vi "sistema_labview.vi"() -> ()   [LabVIEW 2026]
uses:
  <vilib>/Instr/_visa.llb/VISA Flush IO Buffer Mask.ctl
  <vilib>/Instr/_visa.llb/VISA Configure Serial Port (Instr).vi
  tektronix_dpo_mso_2000_4000_series 2/Tektronix DPO MSO 2000 4000 Series/Public/Data/Read (Single Waveform).vi
  <vilib>/express/express analysis/Spectral/Block/exnSpectralBlock spectral measurements RMS poly.vi
  <vilib>/express/express analysis/Spectral/Block/exnSpectralBlock spectral measurements RMS DDT.vi
  <vilib>/express/express analysis/Spectral/XNode/ExpressSpectralMeasurementsBlockNode.xnode
  tektronix_dpo_mso_2000_4000_series 2/Tektronix DPO MSO 2000 4000 Series/Tektronix DPO MSO 2000 4000 Series.lvlib
panel:
  in  "Record":bool
  in  "Filename 2":path=path "test.xlsx" caption="Filename"
  in  "Channel (0: Channel 1)":u16(ring) items=["Channel 1", "Channel 2", "Channel 3", "Channel 4", "Math", "Reference 1", "Reference 2", "Reference 3", "Reference 4"]
  in  "VISA Resource Name 2":refnum<visa-resource-name>
  out "Com Arduino OK":bool
  in  "VISA resource name":refnum<visa-resource-name>
  out "Motor 1 Round":dbl
  out "Motor 2 Round":dbl
  in  "Resolution (passo/mm)":dbl
  in  "Run Beam":bool
  in  "?":bool=TRUE
  out "Axis 2 Offset":dbl
  out "Axis 1 Offset":dbl
  out "Move Motor 1 (x)":dbl=-3.0
  out "Move Motor 2 (z)":dbl=1.0
  out "Scan Loop":u32=9
  out "Imaging Locations (z,x)":dbl[][](array[numeric])=[[5.0, -5.0], [3.0, -5.0], [1.0, -5.0], [-1.0, -5.0], [-3.0, -5.0], [-5.0, -5.0], [-5.0, -3.0], [-3.0, -3.0], [-1.0, -3.0], [1.0, -3.0], [3.0, -3.0], [5.0, -3.0], [5.0, -1.0], [3.0, -1.0], [1.0, -1.0], [-1.0, -1.0], [-3.0, -1.0], [-5.0, -1.0], [-5.0, 1.0], [-3.0, 1.0], [-1.0, 1.0], [1.0, 1.0], [3.0, 1.0], [5.0, 1.0], [5.0, 3.0], [3.0, 3.0], [1.0, 3.0], [-1.0, 3.0], [-3.0, 3.0], [-5.0, 3.0]]
  out "Graph Locations (x,z)":u32[][](array[numeric])
  out "Scanned Data positive":dbl[][](array[numeric])
  out "Scanned Data negative":dbl[][](array[numeric])
  out "Axis 2 Step":dbl=10.0
  out "Axis 1 Step":dbl
  out "Placement":dbl[](array[numeric])
  out "Beam Map Execution (%)":dbl(knob)=0.3 scale=0.0..1.0
  in  "Axis 2 Divisions":u32=5
  in  "Axis 1 Divisions":u32=5
  in  "Axis 1 Distance x(mm)":dbl=10.0
  in  "Axis 2 Distance z(mm)":dbl=10.0
  out "initialized array":dbl[][](array[numeric])
  out "output array":dbl[][](array[numeric])
  out "Intensity Graph":dbl[][](graph)
  out "Z inicial (PACE)":i32
  out "X inicial (PACE)":i32
  in  "X min FFT (kHz)":dbl
  in  "X max FFT (MHz)":dbl=4000.0
  in  "Y max scope (V)":dbl=1.0
  in  "Y min scope (V)":dbl=-1.0
  in  "X max scope (us)":dbl=100.0
  in  "X min scope (us)":dbl
  in  "Lower Cut-Off":dbl=100.0
  in  "Activate Filter":bool
  out "Frequency Spectrum":dynamicdata(graph)
  out "Osciloscopio":dynamicdata(graph)
  in  "offset":dbl
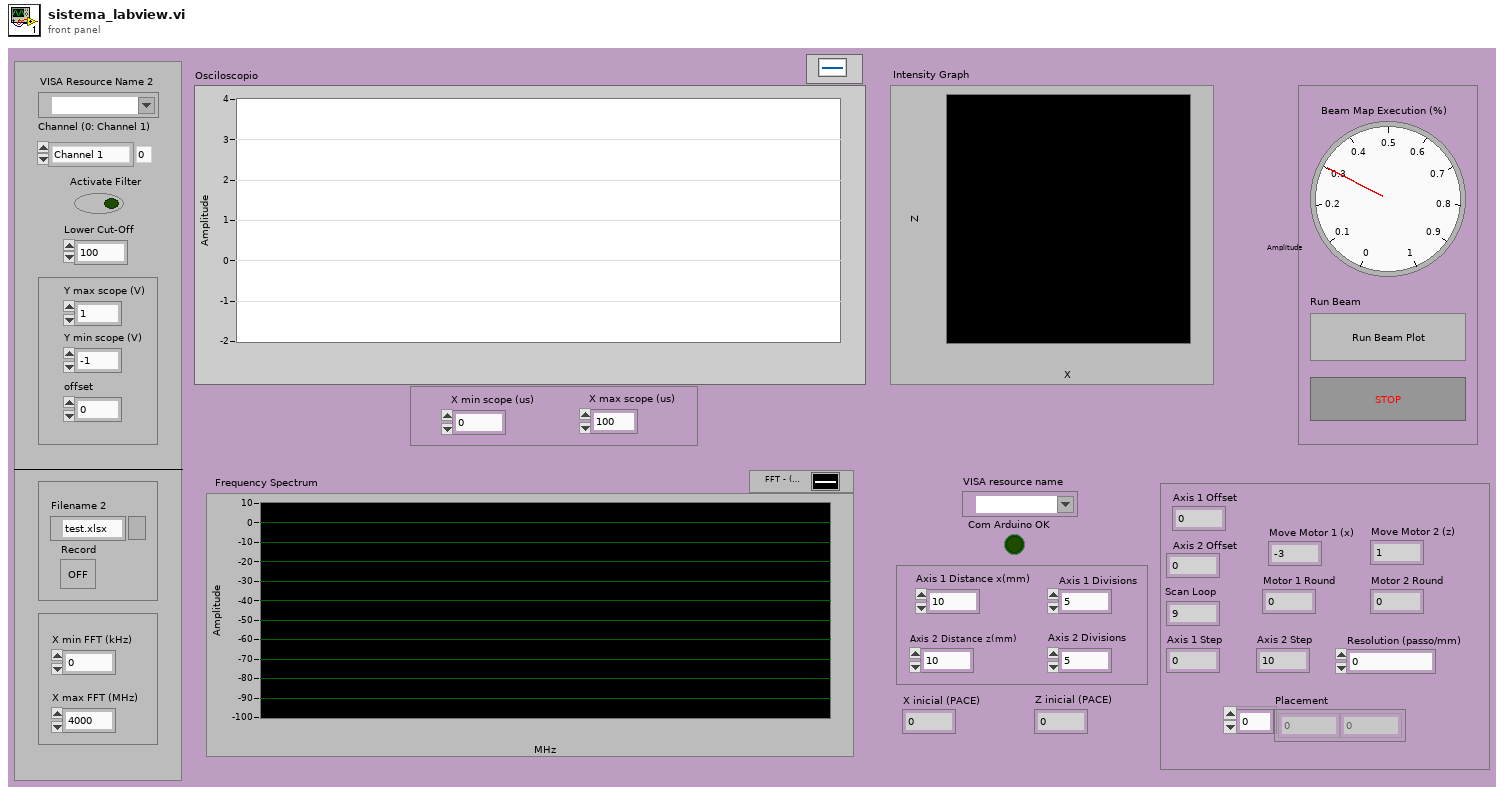
[diagram p1: front panel]
types:
  T1 = typedef "VISA Flush IO Buffer Mask.ctl" = u16
  T2 = cluster{"averaging mode":u16, "weighting mode":u16, "number of averages":u32}
  T3 = cluster{"dB On (F)":bool, "unwrap phase (F)":bool, "convert to degree (F)":bool}
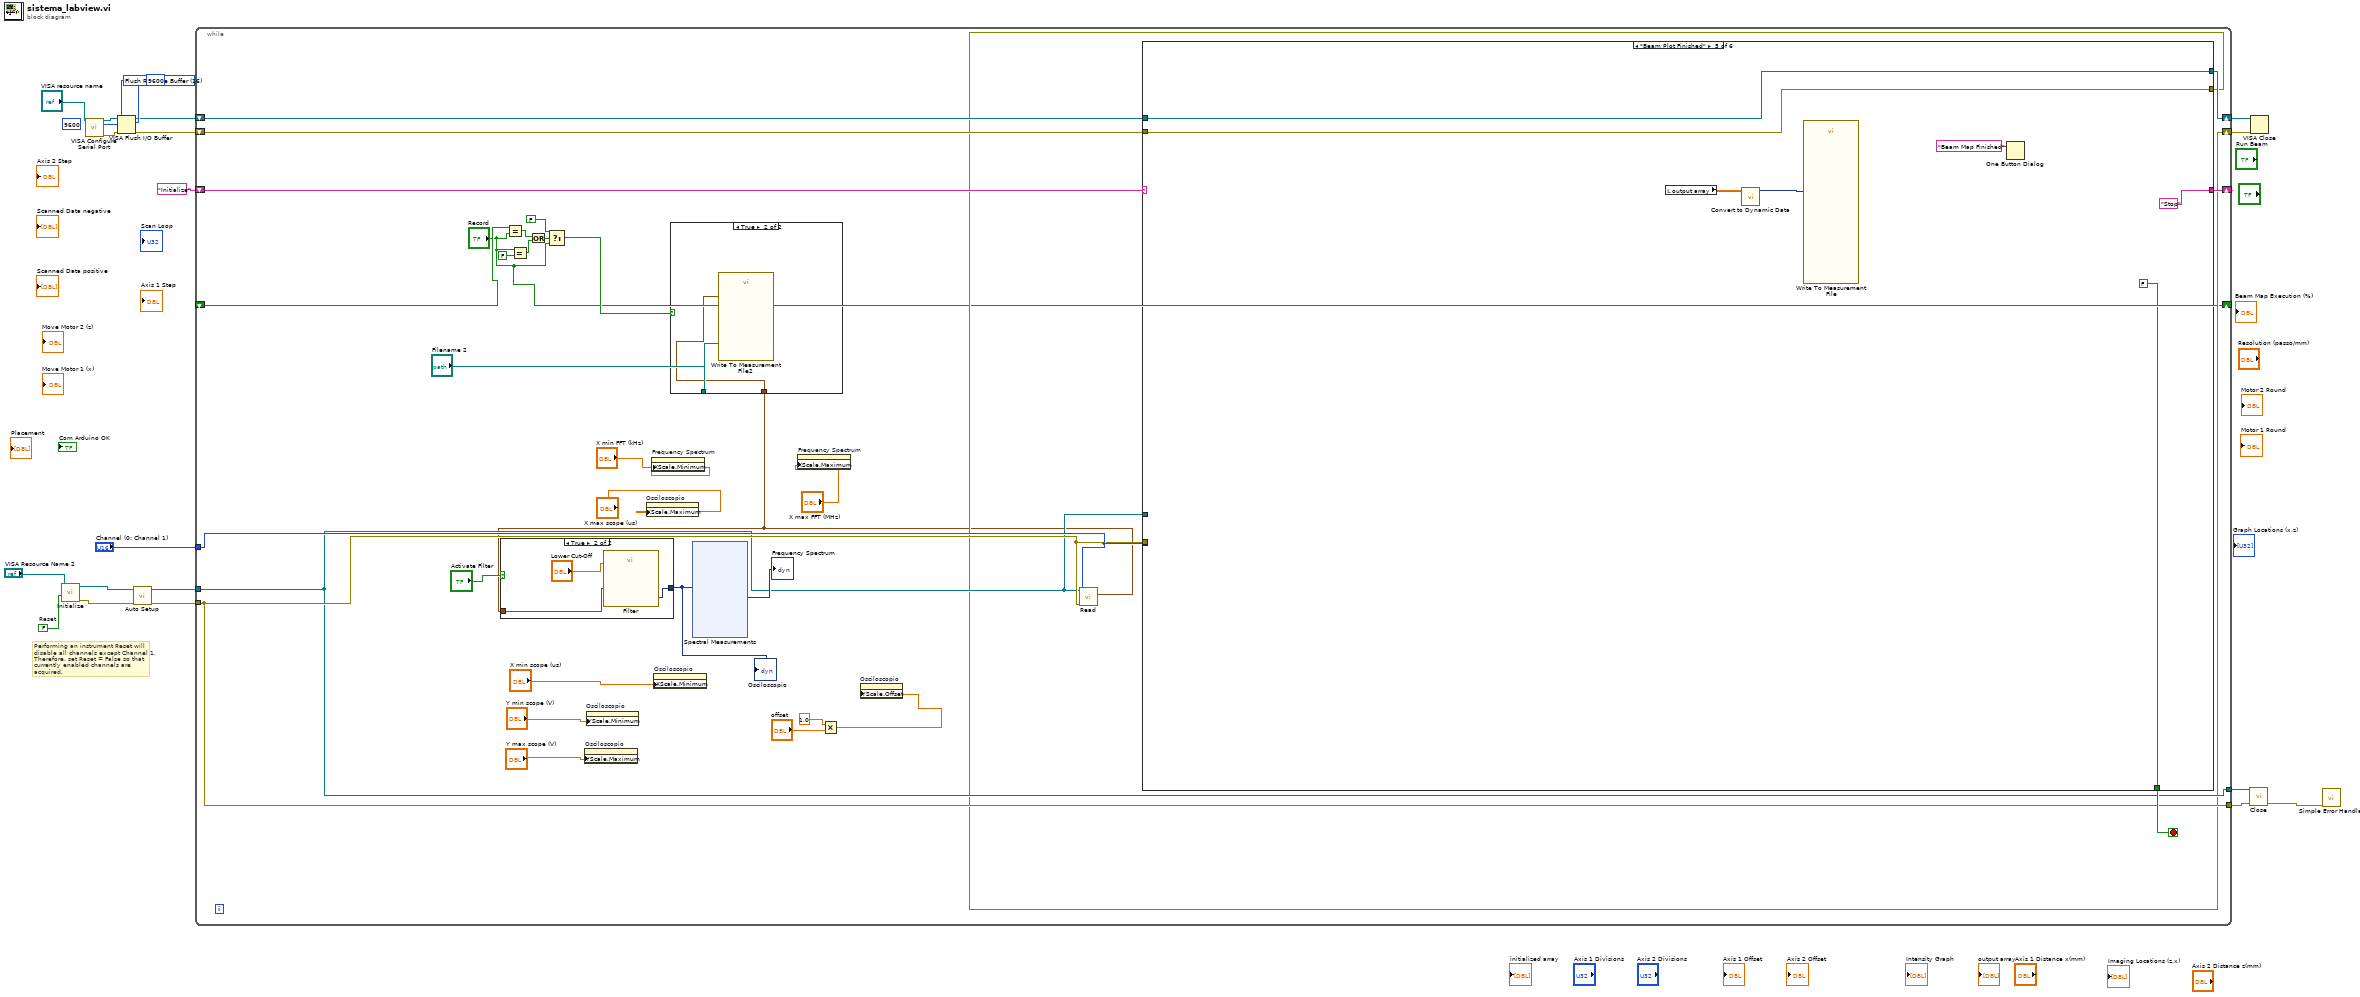
[diagram p0: block diagram]
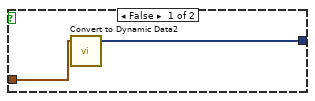
[diagram p3: hidden frame]
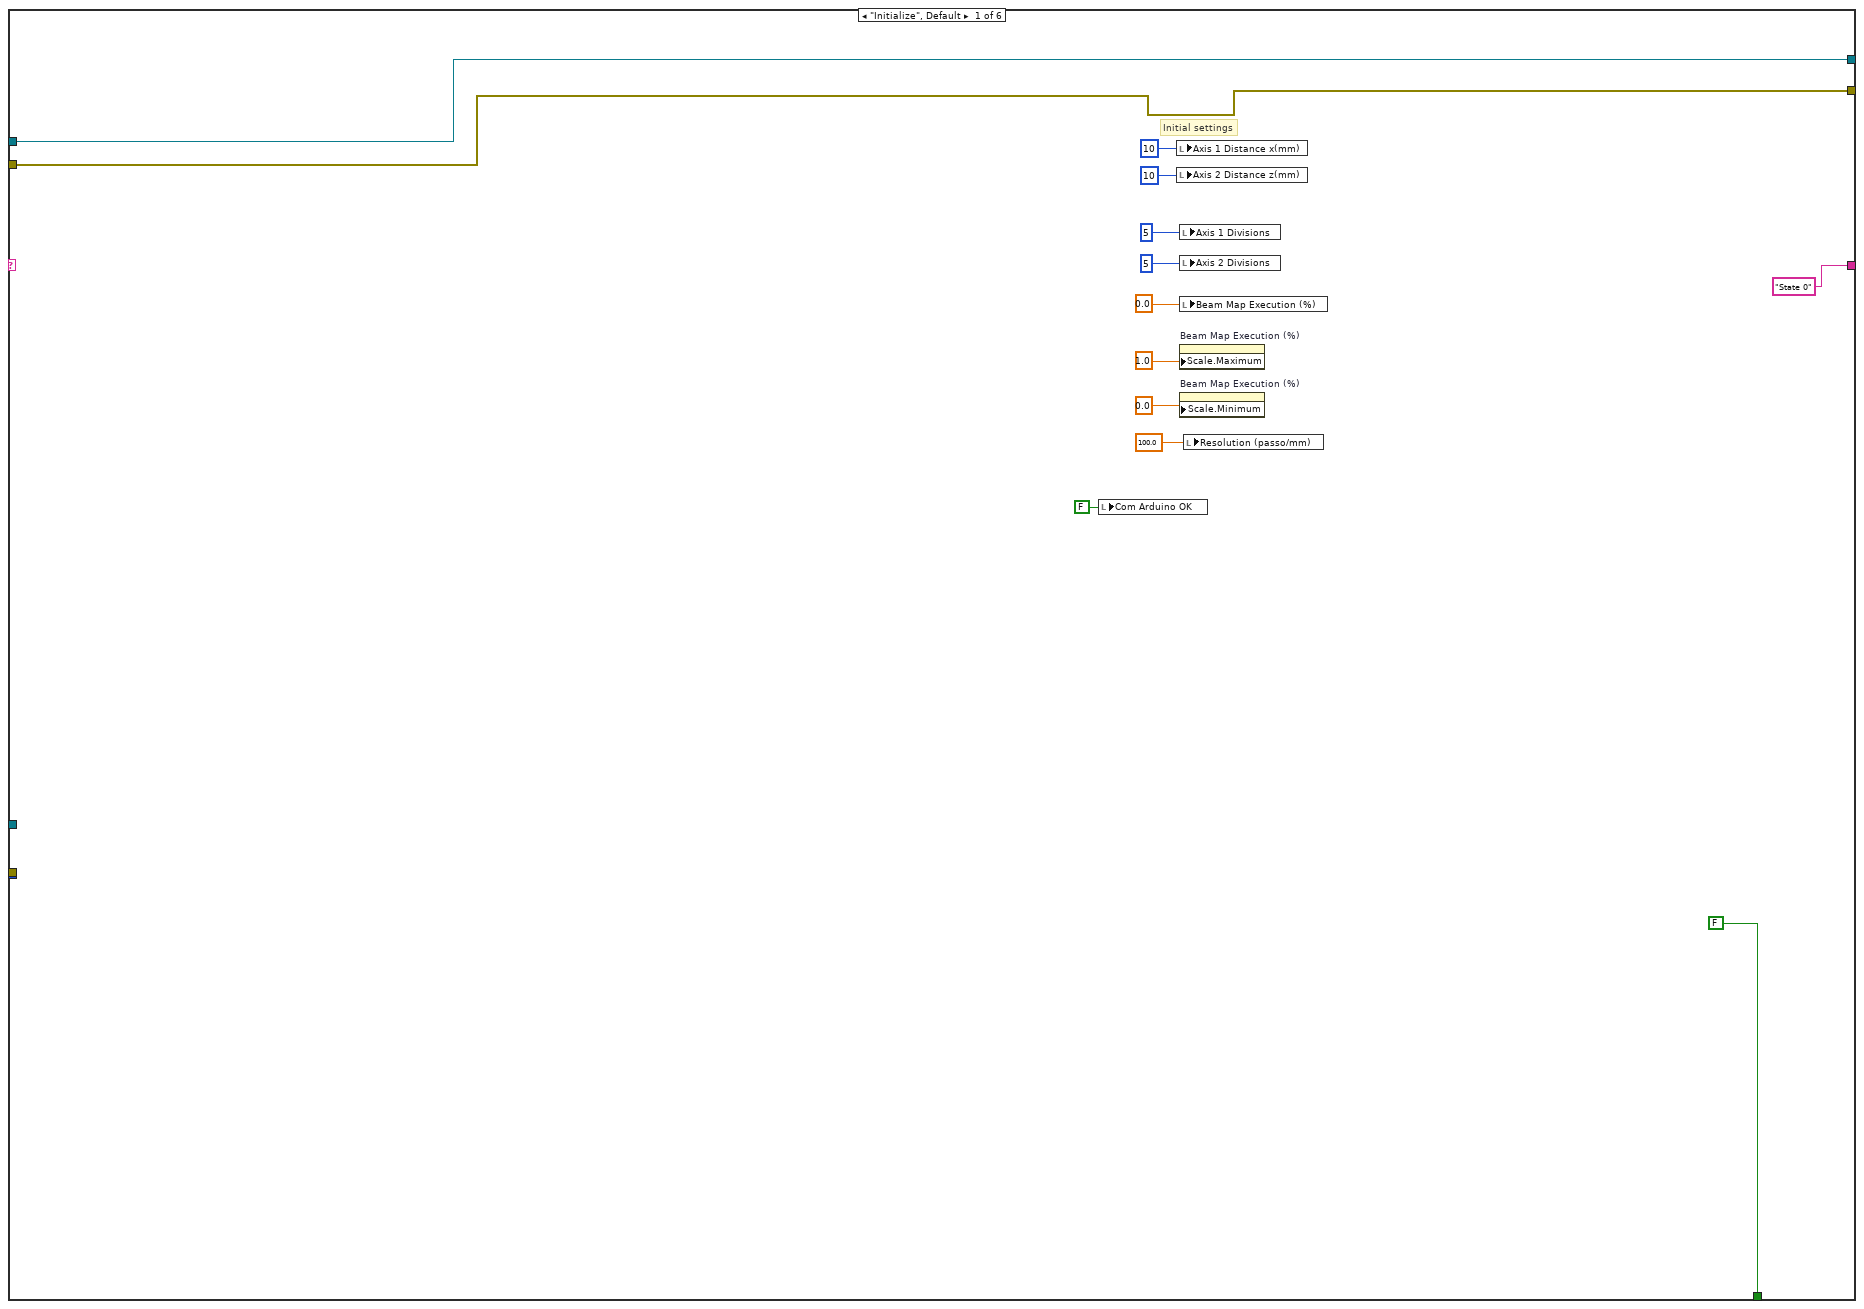
[diagram p4: hidden frame]
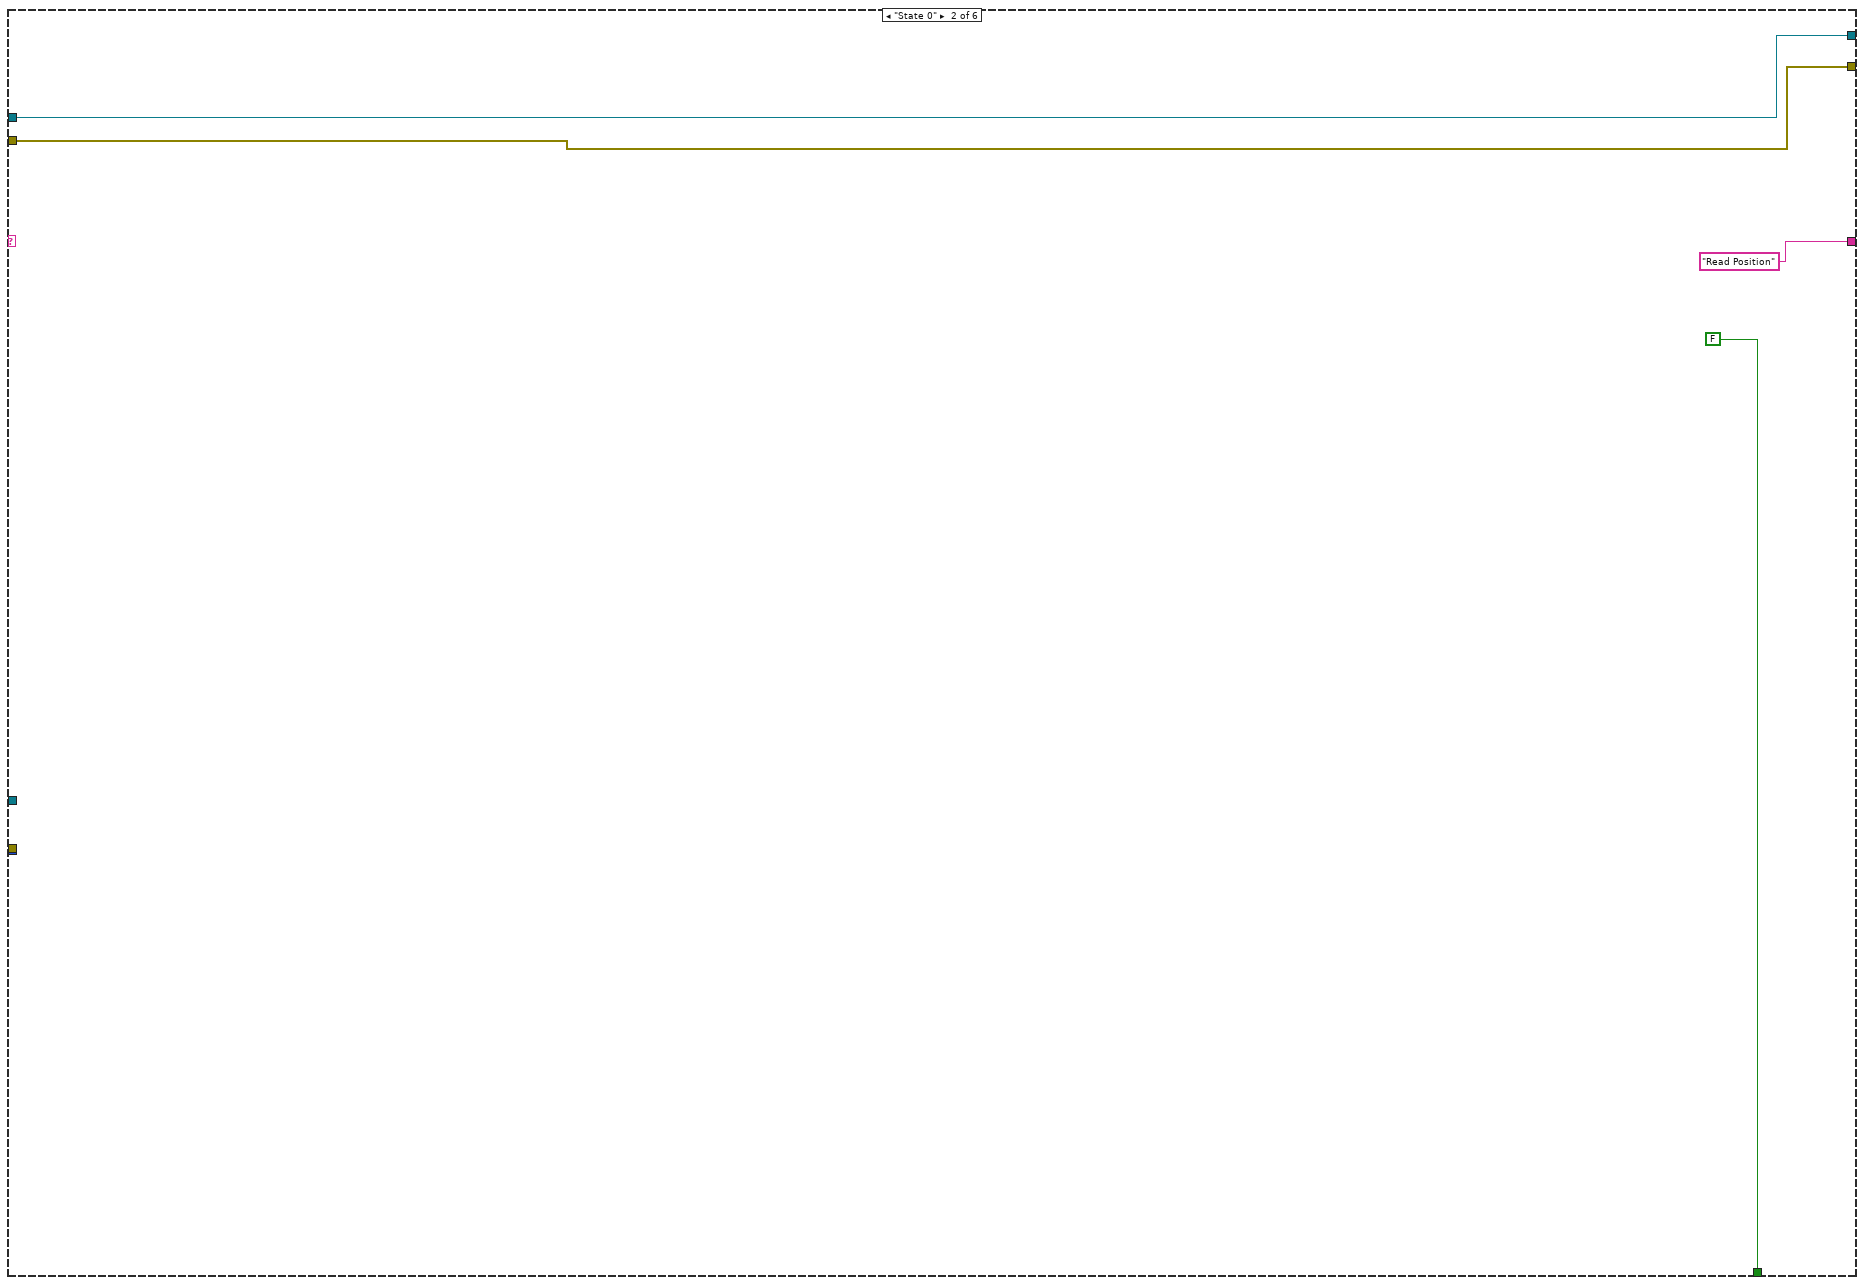
[diagram p5: hidden frame]
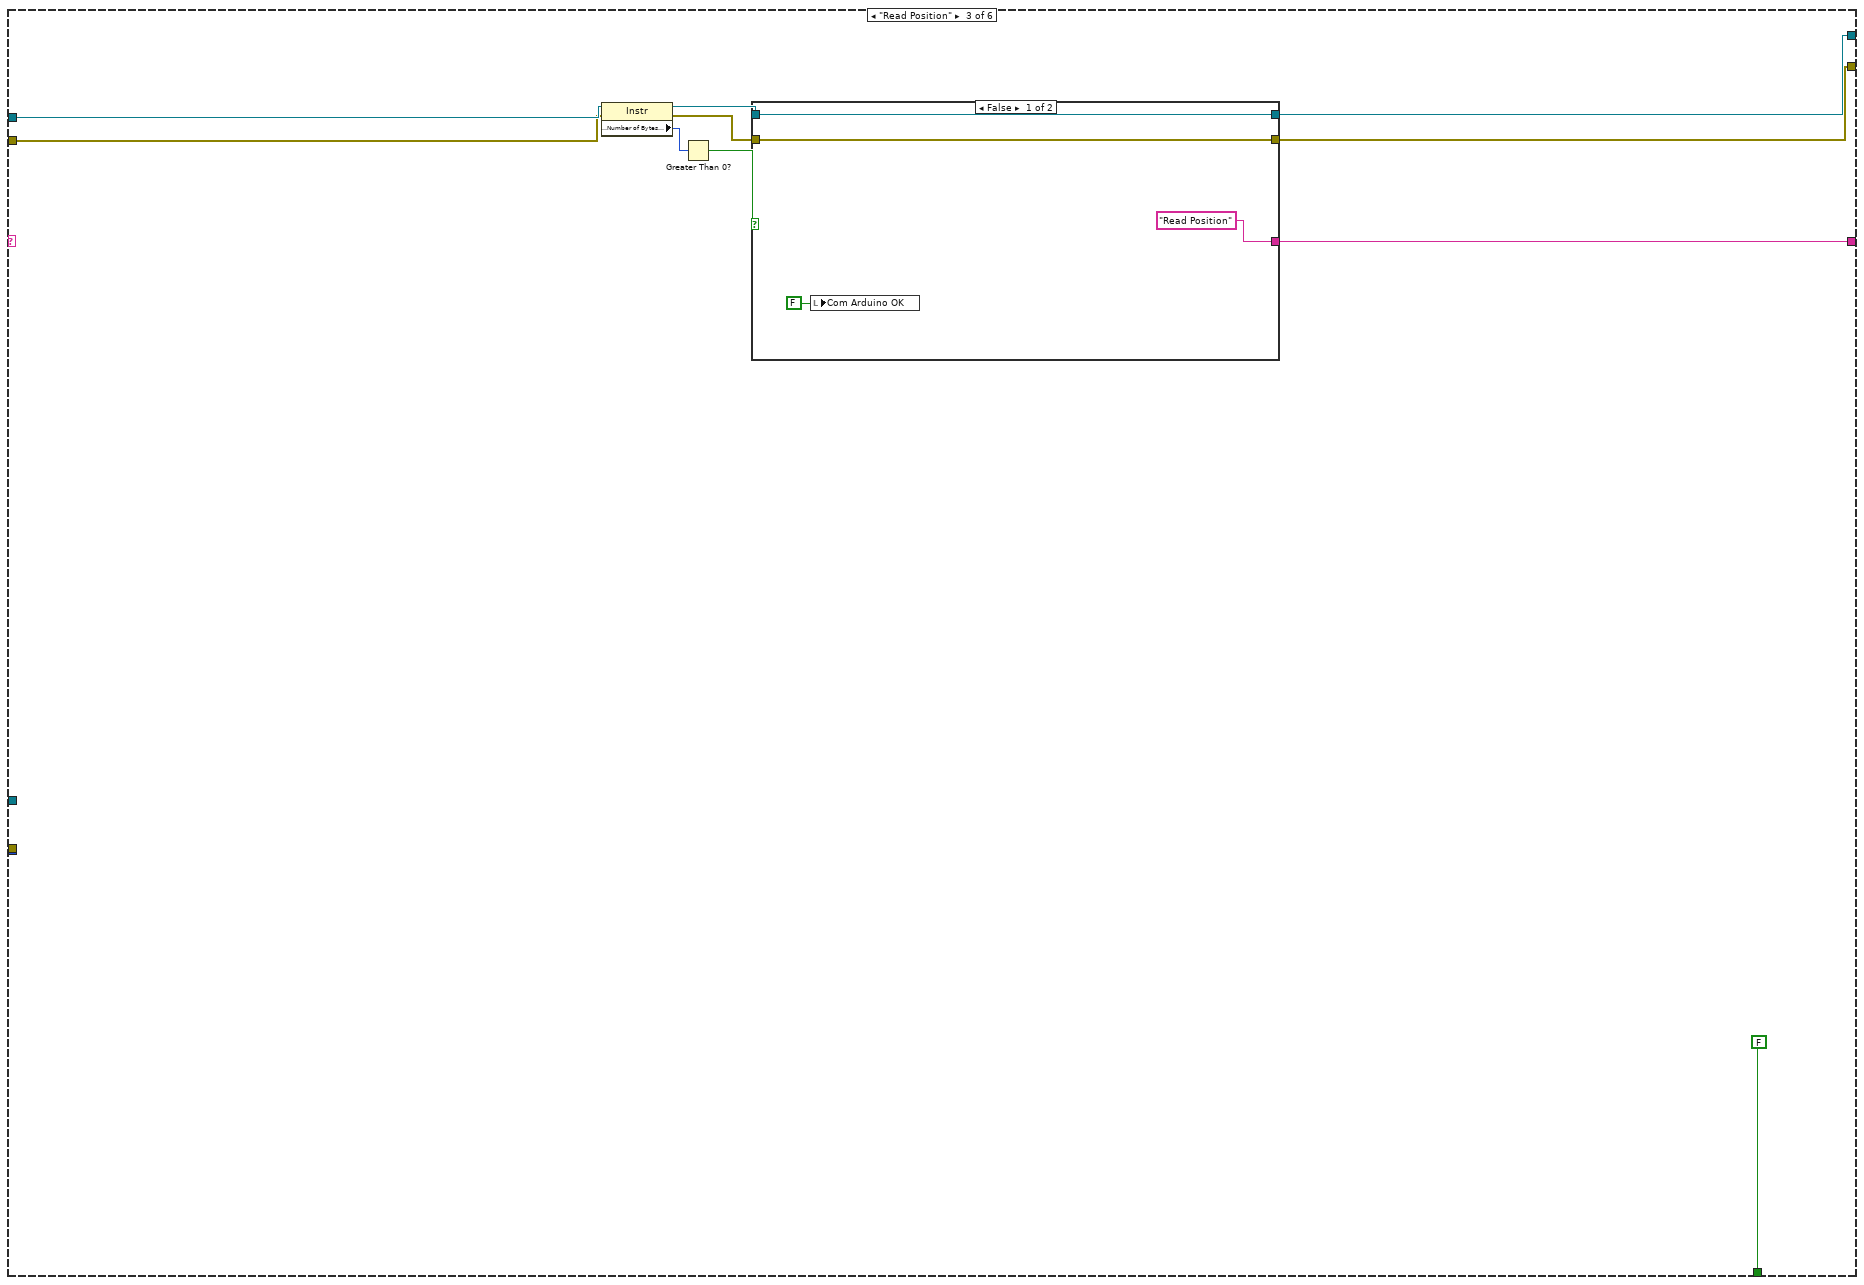
[diagram p6: hidden frame]
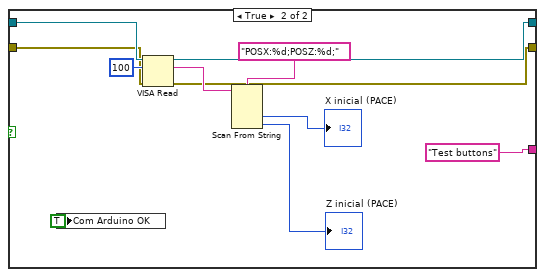
[diagram p7: hidden frame]
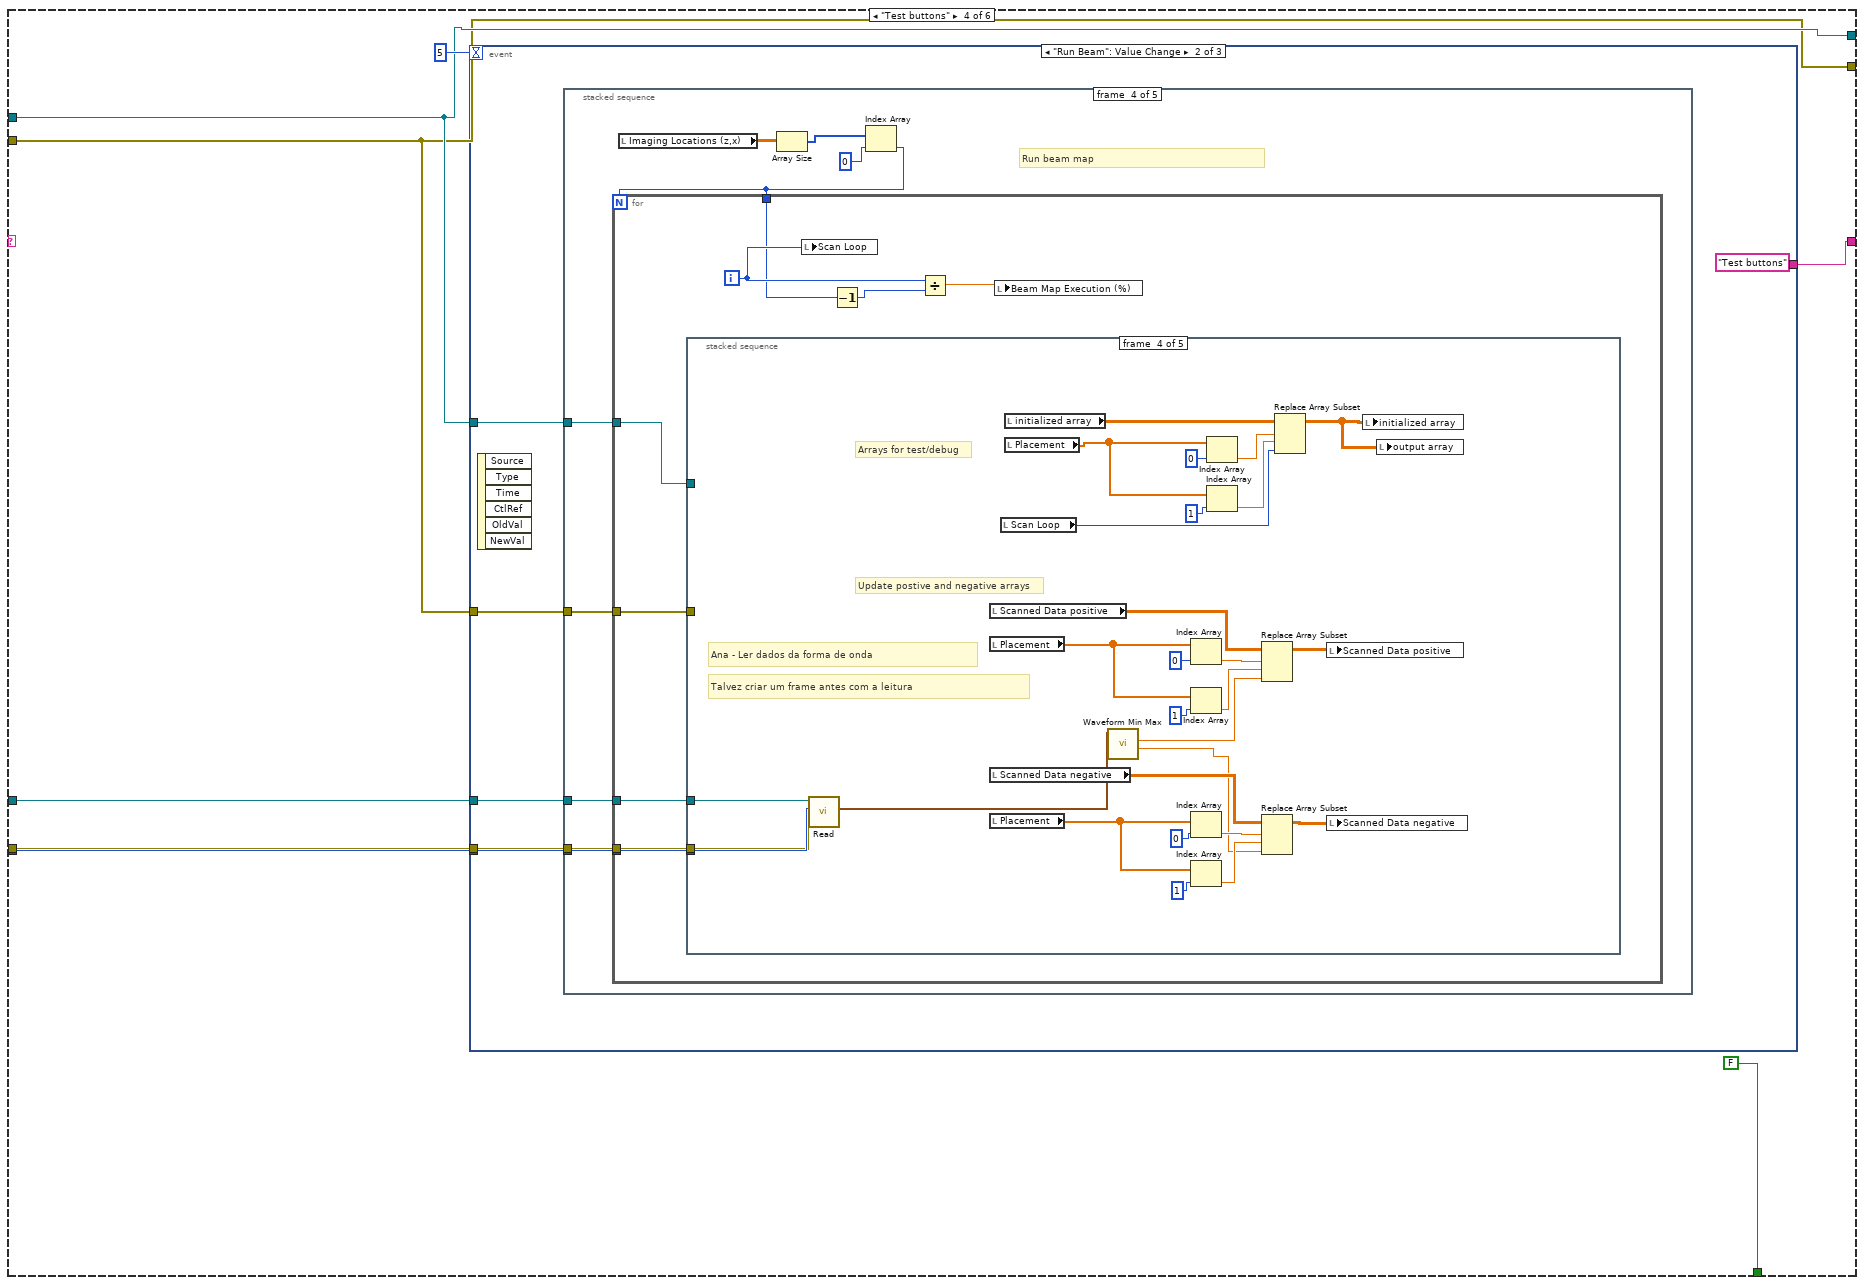
[diagram p8: hidden frame]
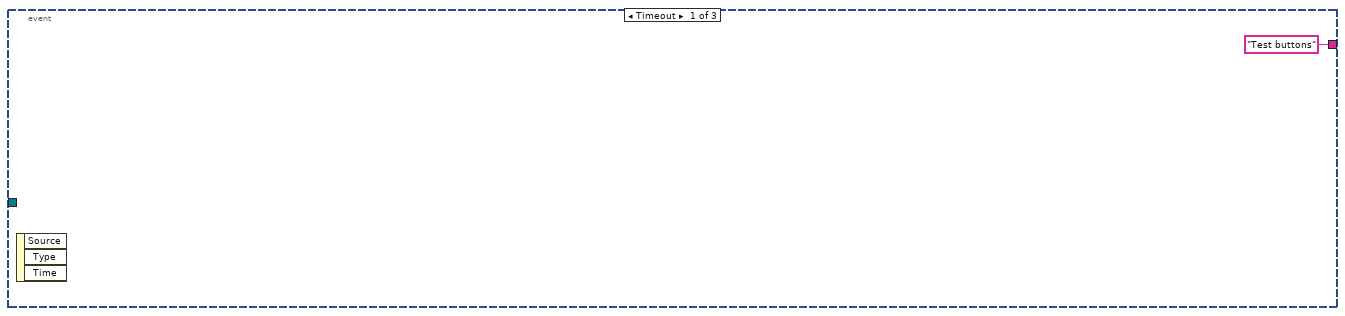
[diagram p9: hidden frame]
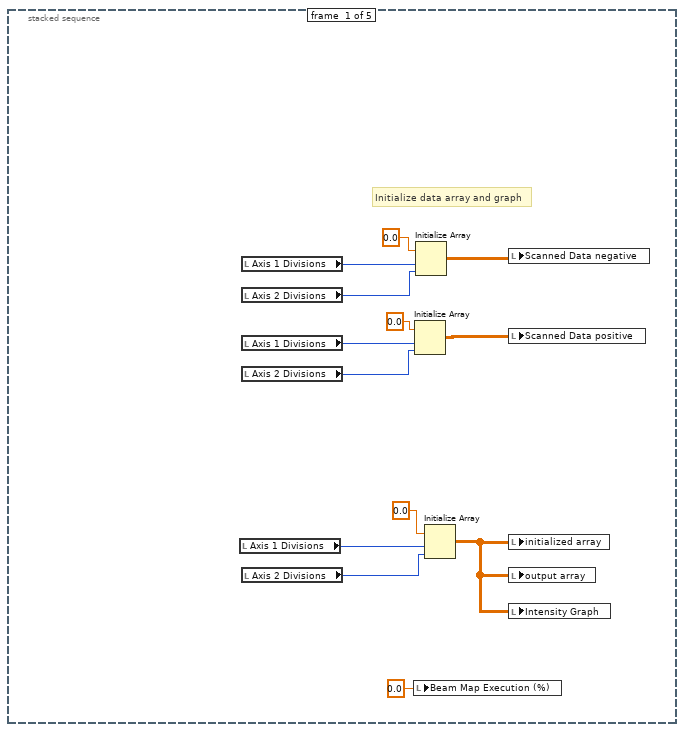
[diagram p10: hidden frame]
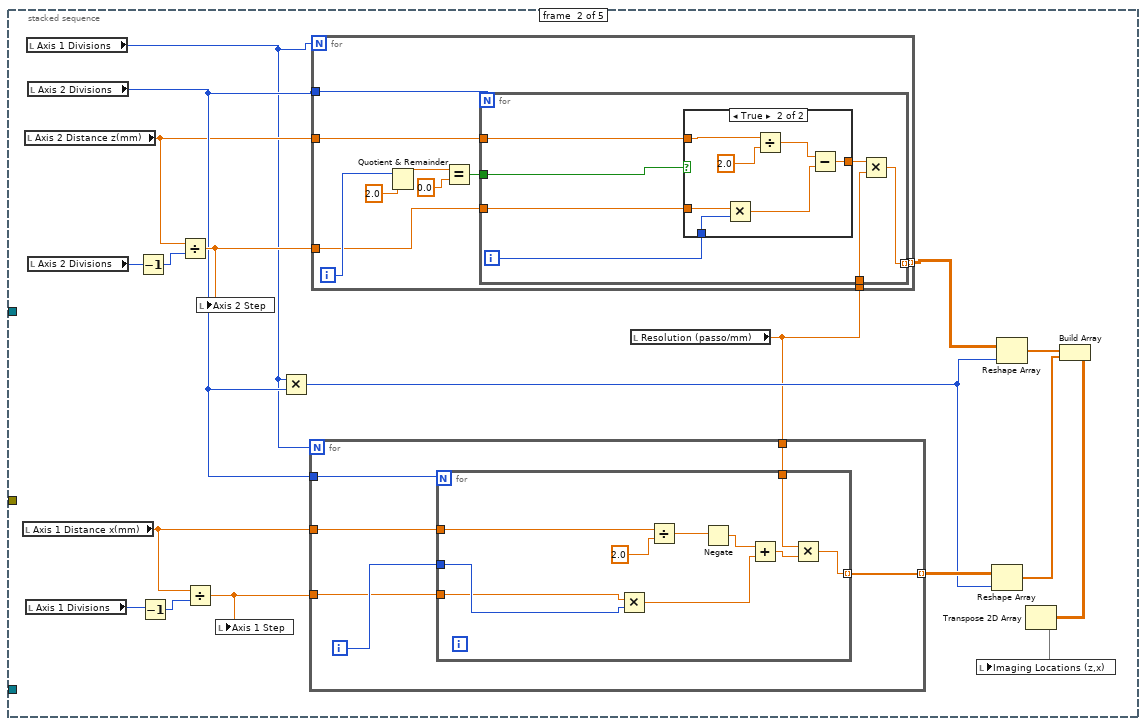
[diagram p11: hidden frame]
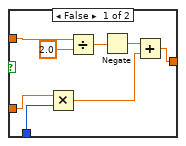
[diagram p12: hidden frame]
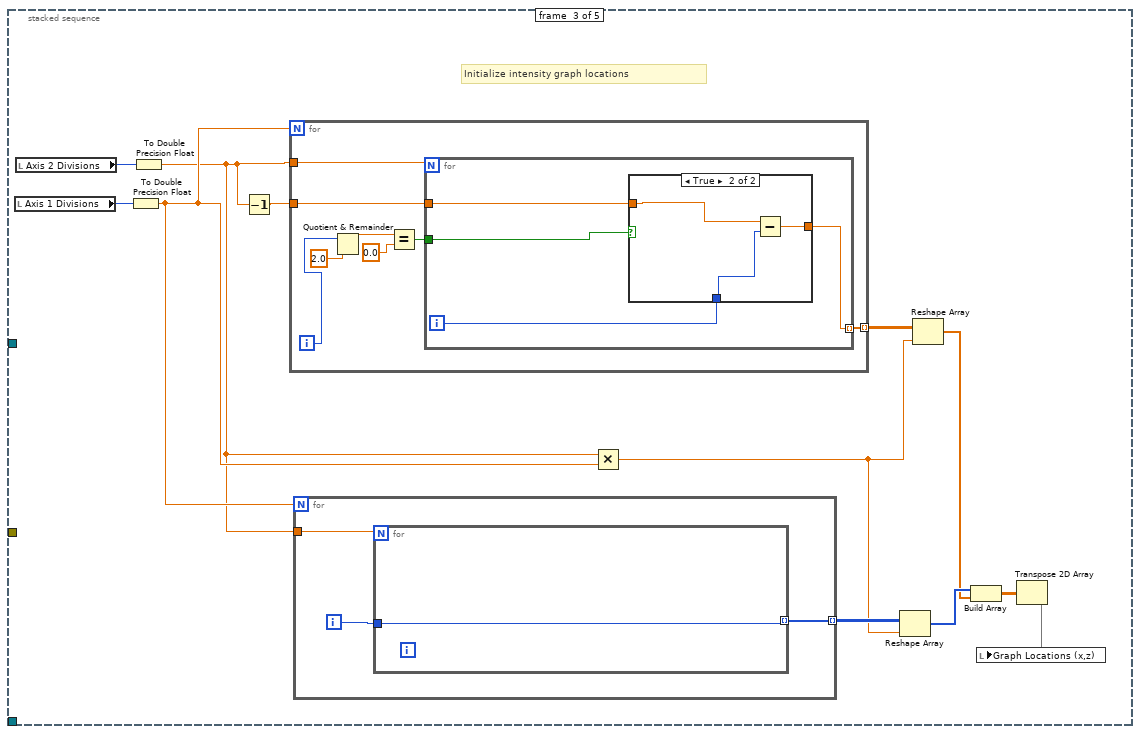
[diagram p13: hidden frame]
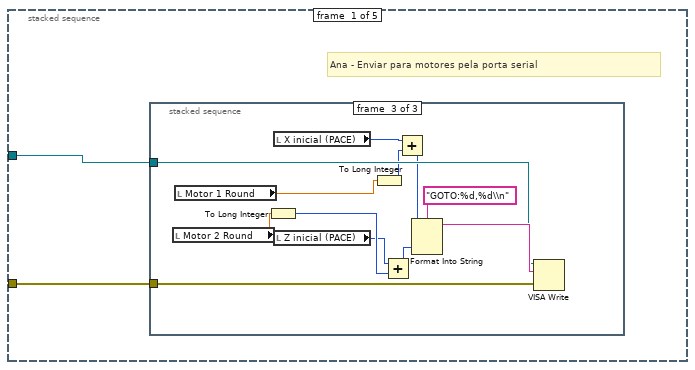
[diagram p15: hidden frame]
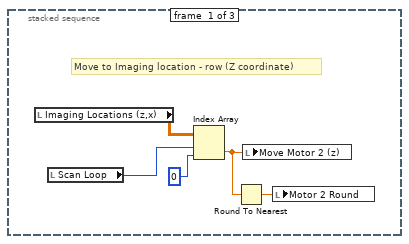
[diagram p16: hidden frame]
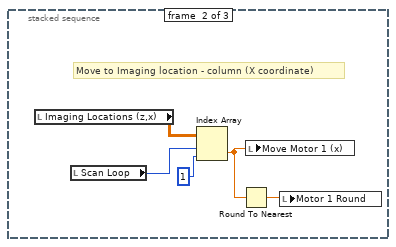
[diagram p17: hidden frame]
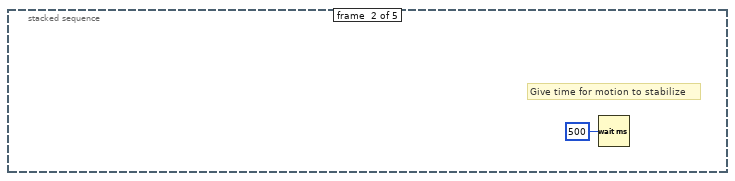
[diagram p18: hidden frame]
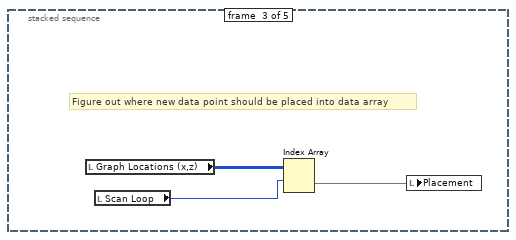
[diagram p19: hidden frame]
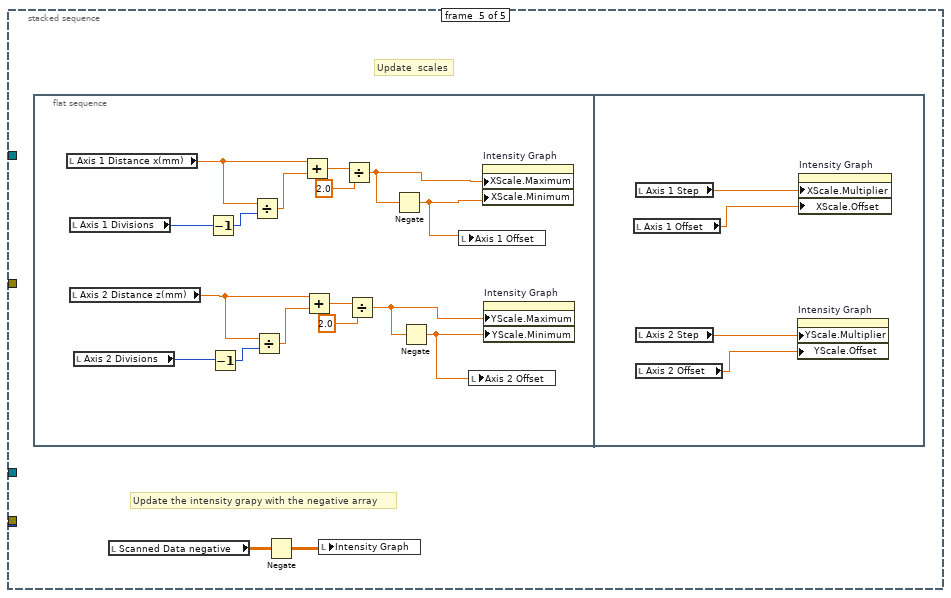
[diagram p20: hidden frame]
diagram:
  w9 = FALSE  # Reset
  (unwired) u32 9600 ("baud rate (9600)")
  w15 = T1 16 items=["Flush Receive Buffer"=16, "Write Transmit Buffer to Device"=32, "Flush Receive Buffer (No I/O)"=64, "Flush Transmit Buffer"=128] ("Mask")
  # "Performing an instrument Reset will disable all channels except Channel 1. Therefore, set Reset = False so that currently enabled channels are acquired."
  n1 = call "Initialize.vi"("Reset (True)"=w9, "VISA resource name"="VISA Resource Name 2") -> ("error out"=w8:errorcluster, "VISA resource name out"=w7:refnum<visa-resource-name>)  [unwired: 8 in]
  n2 = call-poly "VISA Configure Serial Port"("VISA resource name"="VISA resource name", "baud rate (9600)"=u32 9600) -> ("VISA resource name out"=w17:refnum<visa-resource-name>, "error out"=w16:errorcluster)  [unwired: 12 in]
  n3 = VISA Flush I/O Buffer(VISA resource name=w17, mask (16)=w15, error in (no error)=w16) -> (VISA resource name out=w14:refnum<visa-resource-name>, error out=w13:errorcluster)
  n4 = call "Auto Setup.vi"("error in (no error)"=w8, "VISA resource name"=w7) -> ("error out"=w6:errorcluster, "VISA resource name out"=w5:refnum<visa-resource-name>)  [unwired: 8 in]
  n5 = while {
    shift-right: [w52] -> _
    shift-left: "Initialize" -> [w51]
    shift-right: [w49] -> w12
    shift-left: w14 -> [w50]
    shift-right: [w31] -> w11
    shift-left: w13 -> [w48]
    tunnel: w6 -> [w33]
    tunnel: w5 -> [w32]
    tunnel: "Channel (0: Channel 1)" -> [w34]
    tunnel: [w33] -> w2
    tunnel: [w32] -> w1
    shift-right: ["Record"] -> _
    shift-left: _ -> [w23]
    stop <- w35 stop-if-true
    n6 = Equal?(x=w23, y="Record") -> (x = y?=w28:bool)
    n7 = Equal?(x="Record", y=FALSE) -> (x = y?=w27:bool)
    n8 = Or(x=w28, y=w27) -> (x .or. y?=w29:bool)
    n9 = Select(t=FALSE, s=w29, f="Record") -> (s? t:f=w24:bool)
    n10 = property on="Osciloscopio" class="WFGraph (strict)"("YScale.Maximum"="Y max scope (V)") -> ()  [unwired: 2 in, 2 out]
    n11 = property on="Osciloscopio" class="WFGraph (strict)"("YScale.Minimum"="Y min scope (V)") -> ()  [unwired: 2 in, 2 out]
    n12 = property on="Osciloscopio" class="WFGraph (strict)"("XScale.Maximum"="X max scope (us)") -> ()  [unwired: 2 in, 2 out]
    n13 = property on="Frequency Spectrum" class="WFGraph (strict)"("XScale.Minimum"="X min FFT (kHz)") -> ()  [unwired: 2 in, 2 out]
    n14 = property on="Osciloscopio" class="WFGraph (strict)"("XScale.Minimum"="X min scope (us)") -> ()  [unwired: 2 in, 2 out]
    n15 = property on="Frequency Spectrum" class="WFGraph (strict)"("XScale.Maximum"="X max FFT (MHz)") -> ()  [unwired: 2 in, 2 out]
    n16 = Multiply(x=1.0, y="offset") -> (x*y=w37:dbl)
    n17 = property on="Osciloscopio" class="WFGraph (strict)"("YScale.Offset"=w37) -> ()  [unwired: 2 in, 2 out]
    n18 = call-poly "Read.vi"("error in (no error)"=w33, "Channel (0: Channel 1)"=w34, "VISA resource name"=w32) -> ("Waveform Graph"=w21:waveform(dbl))  [unwired: 6 in, 2 out]
    n19 = case shown="True" "Activate Filter" {
      tunnel: [w56 w59] -> w36
      tunnel: w21 -> [w55 w57]
      frame False {
        n20 = call "Convert to Dynamic Data2"("Waveform"=w55) -> ("Dynamic Data Type"=w56:dynamicdata)  [unwired: 3 in]
      }
      frame True {
        n21 = call "Filter"("Lower Cut-Off"="Lower Cut-Off", "Signal"=w57) -> ("Filtered Signal"=w59:dynamicdata)  [unwired: 8 in, 1 out]
      }
    }
    "Osciloscopio" <- w36
    n22 = case shown="True" w24 {
      tunnel: "Filename 2" -> [_ w54]
      tunnel: w21 -> [_ w53]
      frame False {
      }
      frame True {
        n23 = call "Write To Measurement File2"("Signals"=w53, "Filename"=w54) -> ()  [unwired: 15 in, 3 out]
      }
    }
    n24 = xnode "Spectral Measurements"("Signals"=w36) -> ("FFT - (RMS)"=→"Frequency Spectrum":dynamicdata)  [unwired: 1 in, 2 out]
    n25 = case shown="\"Beam Plot Finished\"" w51 {
      selector: w51 -> [_ _ _ _ _ w349]
      tunnel: ["State 0" "Read Position" w87 w118 "Stop" w349] -> w52
      tunnel: [FALSE FALSE FALSE FALSE FALSE TRUE] -> w35
      tunnel: w50 -> [w72 w84 w91 w117 w340 w348]
      tunnel: w48 -> [w71 w83 w90 w116 w341 w347]
      tunnel: [w71 w83 w88 w116 w341 w347] -> w31
      tunnel: [w72 w84 w89 w117 w340 w348] -> w49
      tunnel: w34 -> [_ _ _ w114 _ _]
      tunnel: w33 -> [_ _ _ w113 _ _]
      tunnel: w32 -> [_ _ _ w112 _ _]
      frame "Initialize", Default {
        # "Initial settings"
        n26 = local write "Com Arduino OK"(FALSE ("Com Arduino OK")) -> ()
        n27 = local write "Axis 1 Distance x(mm)"(u32 10 ("Axis 1 Distance (mm)")) -> ()
        n28 = local write "Axis 2 Distance z(mm)"(u32 10 ("Axis 2 Distance (mm)")) -> ()
        n29 = local write "Axis 1 Divisions"(u32 5 ("Axis 1 Divisions")) -> ()
        n30 = local write "Axis 2 Divisions"(u32 5 ("Axis 2 Divisions")) -> ()
        n31 = local write "Beam Map Execution (%)"(0.0 ("Beam Map Execution (%)")) -> ()
        n32 = property on="Beam Map Execution (%)" class="Knob (strict)"("Scale.Maximum"=1.0 ("Scale.Range:Maximum")) -> ()  [unwired: 2 in, 2 out]
        n33 = property on="Beam Map Execution (%)" class="Knob (strict)"("Scale.Minimum"=0.0 ("Scale.Range:Maximum")) -> ()  [unwired: 2 in, 2 out]
        n34 = local write "Resolution (passo/mm)"(100.0 ("Resolution")) -> ()
      }
      frame "State 0" {
      }
      frame "Read Position" {
        n35 = property class="Instr"(reference=w91, error in=w90) -> (reference out=w93:refnum<visa-resource-name>, error out=w92:errorcluster, "Serial Settings:Number of Bytes at Serial Port"=w95:u32)
        n36 = Greater Than 0?(x=w95) -> (x > 0?=w94:bool)
        n37 = case shown="False" w94 {
          tunnel: w93 -> [w100 w106]
          tunnel: w92 -> [w99 w105]
          tunnel: [w100 w104] -> w89
          tunnel: [w99 w103] -> w88
          tunnel: ["Read Position" "Test buttons"] -> w87
          frame False {
            n38 = local write "Com Arduino OK"(FALSE ("Com Arduino OK")) -> ()
          }
          frame True {
            n39 = local write "Com Arduino OK"(TRUE ("Com Arduino OK")) -> ()
            n40 = VISA Read(VISA resource name=w106, byte count=u32 100, error in (no error)=w105) -> (VISA resource name out=w104:refnum<visa-resource-name>, read buffer=w109:string, error out=w103:errorcluster)  [unwired: 1 out]
            n41 = Scan From String(format string="POSX:%d;POSZ:%d;", input string=w109) -> (output 1=→"X inicial (PACE)":i32, output 2=→"Z inicial (PACE)":i32)  [unwired: 4 in, 3 out]
          }
        }
      }
      frame "Test buttons" {
        n42 = event shown="[1] \"Run Beam\": Value Change" {
          selector: _ -> [_ _ _]
          dyn-events: _ -> [_ _ _]
          timeout: 5 -> [_ _ _]
          tunnel: ["Test buttons" "Test buttons" "Stop"] -> w118
          tunnel: w117 -> [_ w125 _]
          tunnel: w116 -> [_ w124 _]
          tunnel: w114 -> [_ w123 _]
          tunnel: w113 -> [_ w122 _]
          tunnel: w112 -> [_ w121 _]
          event Timeout {
            n43 = event-data() -> ()  [unwired: 1 in, 3 out]
          }
          event "Run Beam": Value Change {
            n44 = event-data() -> ()  [unwired: 1 in, 6 out]
            n45 = stacked-sequence {
              tunnel: w125 -> [_ _ _ w242 w334]
              tunnel: w124 -> [_ _ _ w241 _]
              tunnel: w123 -> [_ _ _ w240 _]
              tunnel: w122 -> [_ _ _ w239 _]
              tunnel: w121 -> [_ _ _ w238 _]
              frame #0 {
                # "Initialize data array and graph"
                n46 = local read "Axis 1 Divisions"() -> (w130:u32)
                n47 = local read "Axis 1 Divisions"() -> (w135:u32)
                n48 = local read "Axis 2 Divisions"() -> (w134:u32)
                n49 = local read "Axis 1 Divisions"() -> (w133:u32)
                n50 = local read "Axis 2 Divisions"() -> (w132:u32)
                n51 = local read "Axis 2 Divisions"() -> (w129:u32)
                n52 = local write "Beam Map Execution (%)"(0.0 ("Beam Map Execution (%)")) -> ()
                n53 = Initialize Array(0.0 ("element"), w133, w132) -> (w136:dbl[][])
                n54 = Initialize Array(0.0 ("element"), w135, w134) -> (w137:dbl[][])
                n55 = Initialize Array(0.0, w130, w129) -> (w128:dbl[][])
                n56 = local write "Scanned Data negative"(w137) -> ()
                n57 = local write "Scanned Data positive"(w136) -> ()
                n58 = local write "initialized array"(w128) -> ()
                n59 = local write "output array"(w128) -> ()
                n60 = local write "Intensity Graph"(w128) -> ()
              }
              frame #1 {
                n61 = local read "Axis 1 Distance x(mm)"() -> (w140:dbl)
                n62 = local read "Axis 2 Distance z(mm)"() -> (w142:dbl)
                n63 = local read "Axis 1 Divisions"() -> (w149:u32)
                n64 = local read "Axis 1 Divisions"() -> (w141:u32)
                n65 = local read "Axis 2 Divisions"() -> (w143:u32)
                n66 = local read "Axis 2 Divisions"() -> (w151:u32)
                n67 = Decrement(x=w151) -> (x-1=w150:u32)
                n68 = Decrement(x=w149) -> (x-1=w148:u32)
                n69 = Divide(x=w142, y=w150) -> (x/y=w147:dbl)
                n70 = Divide(x=w140, y=w148) -> (x/y=w146:dbl)
                n71 = local write "Axis 2 Step"(w147) -> ()
                n72 = local write "Axis 1 Step"(w146) -> ()
                n73 = Multiply(x=w141, y=w143) -> (x*y=w152:u32)
                n74 = local read "Resolution (passo/mm)"() -> (w144:dbl)
                n75 = for {
                  N: w141 -> [_]
                  tunnel: [w163] -> w156 mode=indexing
                  tunnel: w143 -> [w162]
                  tunnel: w140 -> [w160]
                  tunnel: w146 -> [w159]
                  tunnel: w144 -> [w158]
                  i -> [w161]
                  n76 = for {
                    N: w162 -> [_]
                    tunnel: [w164] -> w163 mode=indexing
                    tunnel: w161 -> [w171]
                    tunnel: w160 -> [w168]
                    tunnel: w159 -> [w167]
                    tunnel: w158 -> [w165]
                    n77 = Multiply(x=w167, y=w171) -> (x*y=w172:dbl)
                    n78 = Divide(x=w168, y=2.0) -> (x/y=w170:dbl)
                    n79 = Negate(x=w170) -> (-x=w169:dbl)
                    n80 = Add(x=w169, y=w172) -> (x+y=w166:dbl)
                    n81 = Multiply(x=w165, y=w166) -> (x*y=w164:dbl)
                  }
                }
                n82 = for {
                  N: w141 -> [_]
                  tunnel: w143 -> [w183]
                  tunnel: [w182] -> w157 mode=indexing
                  tunnel: w142 -> [w176]
                  tunnel: w147 -> [w175]
                  tunnel: w144 -> [w174]
                  i -> [w177]
                  n83 = Quotient & Remainder(x=w177, y=2.0) -> (x-y*floor(x/y)=w181:dbl)  [unwired: 1 out]
                  n84 = Equal?(x=w181, y=0.0) -> (x = y?=w178:bool)
                  n85 = for {
                    N: w183 -> [_]
                    tunnel: [w185] -> w182 mode=indexing
                    tunnel: w178 -> [w190]
                    tunnel: w176 -> [w188]
                    tunnel: w175 -> [w187]
                    tunnel: w174 -> [w184]
                    i -> [w189]
                    n86 = case shown="True" w190 {
                      tunnel: w188 -> [w198 w203]
                      tunnel: w187 -> [w193 w202]
                      tunnel: w189 -> [w192 w201]
                      tunnel: [w194 w200] -> w186
                      frame False {
                        n87 = Multiply(x=w193, y=w192) -> (x*y=w191:dbl)
                        n88 = Divide(x=w198, y=2.0) -> (x/y=w196:dbl)
                        n89 = Negate(x=w196) -> (-x=w195:dbl)
                        n90 = Add(x=w195, y=w191) -> (x+y=w194:dbl)
                      }
                      frame True {
                        n91 = Multiply(x=w202, y=w201) -> (x*y=w204:dbl)
                        n92 = Divide(x=w203, y=2.0) -> (x/y=w199:dbl)
                        n93 = Subtract(x=w199, y=w204) -> (x-y=w200:dbl)
                      }
                    }
                    n94 = Multiply(x=w186, y=w184) -> (x*y=w185:dbl)
                  }
                }
                n95 = Reshape Array(w156, w152) -> (w154:dbl[])
                n96 = Reshape Array(w157, w152) -> (w155:dbl[])
                n97 = Build Array(w155, w154) -> (w153:dbl[][])
                n98 = Transpose 2D Array(2D array=w153) -> (transposed array=w145:dbl[][])
                n99 = local write "Imaging Locations (z,x)"(w145) -> ()
              }
              frame #2 {
                # "Initialize intensity graph locations"
                n100 = local read "Axis 1 Divisions"() -> (w210:u32)
                n101 = local read "Axis 2 Divisions"() -> (w208:u32)
                n102 = To Double Precision Float(number=w210) -> (double precision float=w209:dbl)
                n103 = To Double Precision Float(number=w208) -> (double precision float=w206:dbl)
                n104 = Decrement(x=w206) -> (x-1=w207:dbl)
                n105 = for {
                  N: w209 -> [_]
                  tunnel: w206 -> [w229]
                  tunnel: [w228] -> w216 mode=indexing
                  tunnel: w207 -> [w222]
                  i -> [w223]
                  n106 = Quotient & Remainder(x=w223, y=2.0) -> (x-y*floor(x/y)=w227:dbl)  [unwired: 1 out]
                  n107 = Equal?(x=w227, y=0.0) -> (x = y?=w224:bool)
                  n108 = for {
                    N: w229 -> [_]
                    tunnel: [w233] -> w228 mode=indexing
                    tunnel: w224 -> [w232]
                    tunnel: w222 -> [w230]
                    i -> [w231]
                    n109 = case shown="True" w232 {
                      tunnel: w230 -> [_ w235]
                      tunnel: w231 -> [w234 w236]
                      tunnel: [w234 w237] -> w233
                      frame False {
                      }
                      frame True {
                        n110 = Subtract(x=w235, y=w236) -> (x-y=w237:dbl)
                      }
                    }
                  }
                }
                n111 = for {
                  N: w209 -> [_]
                  tunnel: w206 -> [w220]
                  tunnel: [w219] -> w215 mode=indexing
                  i -> [w218]
                  n112 = for {
                    N: w220 -> [_]
                    tunnel: [w221] -> w219 mode=indexing
                    tunnel: w218 -> [w221]
                  }
                }
                n113 = Multiply(x=w206, y=w209) -> (x*y=w214:dbl)
                n114 = Reshape Array(w215, w214) -> (w212:i32[])
                n115 = Reshape Array(w216, w214) -> (w211:dbl[])
                n116 = Build Array(w212, w211) -> (w217:dbl[][])
                n117 = Transpose 2D Array(2D array=w217) -> (transposed array=w213:dbl[][])
                n118 = local write "Graph Locations (x,z)"(w213) -> ()
              }
              frame #3 {
                # "Run beam map"
                n119 = local read "Imaging Locations (z,x)"() -> (w244:dbl[][])
                n120 = Array Size(array=w244) -> (size(s)=w246:i32[])
                n121 = Index Array "Index Array"(array=w246, index=0) -> (element=w243:i32)
                n122 = for {
                  N: w243 -> [_]
                  tunnel: w243 -> [w252]
                  tunnel: w242 -> [w251]
                  tunnel: w241 -> [w250]
                  tunnel: w240 -> [w249]
                  tunnel: w239 -> [w248]
                  tunnel: w238 -> [w247]
                  i -> [w254]
                  n123 = stacked-sequence {
                    tunnel: w251 -> [w257 _ _ _ _]
                    tunnel: w250 -> [w256 _ _ _ _]
                    tunnel: w249 -> [_ _ _ w287 _]
                    tunnel: w248 -> [_ _ _ w286 _]
                    tunnel: w247 -> [_ _ _ w285 _]
                    frame #0 {
                      # "Ana - Enviar para motores pela porta serial"
                      n124 = stacked-sequence {
                        tunnel: w257 -> [_ _ w275]
                        tunnel: w256 -> [_ _ w268]
                        frame #0 {
                          # "Move to Imaging location - row (Z coordinate)"
                          n125 = local read "Imaging Locations (z,x)"() -> (w262:dbl[][])
                          n126 = local read "Scan Loop"() -> (w261:u32)
                          n127 = Index Array(array=w262, index (row)=w261, index (col)=0 ("disabled index (col)")) -> (element=w258:dbl)
                          n128 = Round To Nearest(number=w258) -> (nearest integer value=w259:dbl)
                          n129 = local write "Move Motor 2 (z)"(w258) -> ()
                          n130 = local write "Motor 2 Round"(w259) -> ()
                        }
                        frame #1 {
                          # "Move to Imaging location - column (X coordinate)"
                          n131 = local read "Imaging Locations (z,x)"() -> (w267:dbl[][])
                          n132 = local read "Scan Loop"() -> (w266:u32)
                          n133 = Index Array(array=w267, index (row)=w266, index (col)=1 ("disabled index (col)")) -> (element=w264:dbl)
                          n134 = Round To Nearest(number=w264) -> (nearest integer value=w263:dbl)
                          n135 = local write "Move Motor 1 (x)"(w264) -> ()
                          n136 = local write "Motor 1 Round"(w263) -> ()
                        }
                        frame #2 {
                          n137 = local read "Motor 2 Round"() -> (w276:dbl)
                          n138 = local read "Motor 1 Round"() -> (w277:dbl)
                          n139 = To Long Integer(number=w276) -> (32bit integer=w271:i32)
                          n140 = local read "X inicial (PACE)"() -> (w274:i32)
                          n141 = local read "Z inicial (PACE)"() -> (w270:i32)
                          n142 = To Long Integer(number=w277) -> (32bit integer=w273:i32)
                          n143 = Add(x=w270, y=w271) -> (x+y=w269:i32)
                          n144 = Add(x=w274, y=w273) -> (x+y=w272:i32)
                          n145 = Format Into String(format string="GOTO:%d,%d\\n", w272, w269) -> (resulting string=w278:string)  [unwired: 2 in, 1 out]
                          n146 = VISA Write(VISA resource name=w275, write buffer=w278, error in (no error)=w268) -> ()  [unwired: 3 out]
                        }
                      }
                    }
                    frame #1 {
                      # "Give time for motion to stabilize"
                      n147 = Wait (ms)(milliseconds to wait=u32 500) -> ()  [unwired: 1 out]
                    }
                    frame #2 {
                      # "Figure out where new data point should be placed into data array"
                      n148 = local read "Graph Locations (x,z)"() -> (w283:u32[][])
                      n149 = local read "Scan Loop"() -> (w282:u32)
                      n150 = Index Array(array=w283, index (row)=w282) -> (element=w281:u32[])  [unwired: 1 in]
                      n151 = local write "Placement"(w281) -> ()
                    }
                    frame #3 {
                      # "Talvez criar um frame antes com a leitura"
                      # "Ana - Ler dados da forma de onda"
                      # "Update postive and negative arrays"
                      # "Arrays for test/debug"
                      n152 = call-poly "Read.vi"("error in (no error)"=w286, "Channel (0: Channel 1)"=w287, "VISA resource name"=w285) -> ("Waveform Graph"=w284:waveform(dbl))  [unwired: 6 in, 2 out]
                      n153 = local read "Scanned Data positive"() -> (w306:dbl[][])
                      n154 = local read "Placement"() -> (w293:dbl[])
                      n155 = local read "Scanned Data negative"() -> (w311:dbl[][])
                      n156 = local read "Placement"() -> (w292:dbl[])
                      n157 = local read "Scan Loop"() -> (w290:u32)
                      n158 = local read "initialized array"() -> (w294:dbl[][])
                      n159 = local read "Placement"() -> (w291:dbl[])
                      n160 = call <vilib>:"Waveform Min Max.vi"("waveform in"=w284) -> ("Y min"=w288:dbl, "Y max"=w289:dbl)  [unwired: 5 in, 4 out]
                      n161 = Index Array(array=w293, index=0) -> (element=w307:dbl)
                      n162 = Index Array(array=w293, index=1 ("disabled index (col)")) -> (element=w308:dbl)
                      n163 = Index Array(array=w292, index=0) -> (element=w310:dbl)
                      n164 = Index Array(array=w292, index=1 ("disabled index (col)")) -> (element=w309:dbl)
                      n165 = Index Array(array=w291, index=0) -> (element=w296:dbl)
                      n166 = Index Array(array=w291, index=1 ("disabled index (col)")) -> (element=w295:dbl)
                      n167 = Replace Array Subset(array=w306, new element=w289, index (row)=w307, index (col)=w308) -> (w302:dbl[][])
                      n168 = Replace Array Subset(array=w311, new element=w288, index (row)=w310, index (col)=w309) -> (w301:dbl[][])
                      n169 = Replace Array Subset(array=w294, new element=w290, index (row)=w296, index (col)=w295) -> (w299:dbl[][])
                      n170 = local write "Scanned Data positive"(w302) -> ()
                      n171 = local write "Scanned Data negative"(w301) -> ()
                      n172 = local write "initialized array"(w299) -> ()
                      n173 = local write "output array"(w299) -> ()
                    }
                    frame #4 {
                      # "Update  scales"
                      # "Update the intensity grapy with the negative array"
                      n174 = flat-sequence {
                        frame #0 {
                          n175 = local read "Axis 1 Distance x(mm)"() -> (w327:dbl)
                          n176 = local read "Axis 1 Divisions"() -> (w329:u32)
                          n177 = local read "Axis 2 Distance z(mm)"() -> (w322:dbl)
                          n178 = local read "Axis 2 Divisions"() -> (w323:u32)
                          n179 = Decrement(x=w329) -> (x-1=w328:u32)
                          n180 = Decrement(x=w323) -> (x-1=w325:u32)
                          n181 = Divide(x=w327, y=w328) -> (x/y=w326:dbl)
                          n182 = Divide(x=w322, y=w325) -> (x/y=w324:dbl)
                          n183 = Add(x=w327, y=w326) -> (x+y=w321:dbl)
                          n184 = Add(x=w322, y=w324) -> (x+y=w318:dbl)
                          n185 = Divide(x=w321, y=2.0) -> (x/y=w317:dbl)
                          n186 = Divide(x=w318, y=2.0) -> (x/y=w315:dbl)
                          n187 = Negate(x=w317) -> (-x=w316:dbl)
                          n188 = Negate(x=w315) -> (-x=w314:dbl)
                          n189 = local write "Axis 1 Offset"(w316) -> ()
                          n190 = local write "Axis 2 Offset"(w314) -> ()
                          n191 = property on="Intensity Graph" class="IntGraph (strict)"("XScale.Maximum"=w317, "XScale.Minimum"=w316) -> ()  [unwired: 2 in, 2 out]
                          n192 = property on="Intensity Graph" class="IntGraph (strict)"("YScale.Maximum"=w315, "YScale.Minimum"=w314) -> ()  [unwired: 2 in, 2 out]
                        }
                        frame #1 {
                          n193 = local read "Axis 1 Offset"() -> (w331:dbl)
                          n194 = local read "Axis 1 Step"() -> (w333:dbl)
                          n195 = local read "Axis 2 Step"() -> (w332:dbl)
                          n196 = local read "Axis 2 Offset"() -> (w330:dbl)
                          n197 = property on="Intensity Graph" class="IntGraph (strict)"("YScale.Multiplier"=w332, "YScale.Offset"=w330) -> ()  [unwired: 2 in, 2 out]
                          n198 = property on="Intensity Graph" class="IntGraph (strict)"("XScale.Multiplier"=w333, "XScale.Offset"=w331) -> ()  [unwired: 2 in, 2 out]
                        }
                      }
                      n199 = local read "Scanned Data negative"() -> (w313:dbl[][])
                      n200 = Negate(x=w313) -> (-x=w312:dbl[][])
                      n201 = local write "Intensity Graph"(w312) -> ()
                    }
                  }
                  n202 = local write "Scan Loop"(w254) -> ()
                  n203 = Decrement(x=w252) -> (x-1=w253:i32)
                  n204 = Divide(x=w254, y=w253) -> (x/y=w255:dbl)
                  n205 = local write "Beam Map Execution (%)"(w255) -> ()
                }
              }
              frame #4 {
                n206 = local read "X inicial (PACE)"() -> (w338:i32)
                n207 = local read "Z inicial (PACE)"() -> (w337:i32)
                n208 = Format Into String(format string="GOTO:%d,%d\\n", w338, w337) -> (resulting string=w335:string)  [unwired: 2 in, 1 out]
                n209 = VISA Write(VISA resource name=w334, write buffer=w335) -> ()  [unwired: 1 in, 3 out]
              }
            }
          }
          event Value Change {
            n210 = event-data() -> ()  [unwired: 1 in, 6 out]
          }
        }
      }
      frame "Beam Plot Finished" {
        n211 = local read "output array"() -> (w343:dbl[][])
        n212 = call "Convert to Dynamic Data"("2D Array"=w343) -> ("Dynamic Data Type"=w342:dynamicdata)  [unwired: 3 in]
        n213 = call "Write To Measurement File"("Signals"=w342) -> ()  [unwired: 16 in, 3 out]
        n214 = One Button Dialog(message="Beam Map Finished") -> ()  [unwired: 1 in, 1 out]
      }
      frame "Stop" {
      }
    }
  }
  n215 = call "Close.vi"("error in (no error)"=w2, "VISA resource name"=w1) -> ("error out"=w3:errorcluster)  [unwired: 9 in]
  n216 = VISA Close(VISA resource name=w12, error in (no error)=w11) -> ()  [unwired: 1 out]
  n217 = call <vilib>:"Simple Error Handler.vi"("error in (no error)"=w3) -> ()  [unwired: 4 in, 5 out]
